vi "about.vi"() -> ()   [LabVIEW 2014]
panel:
  out "专利信息":string
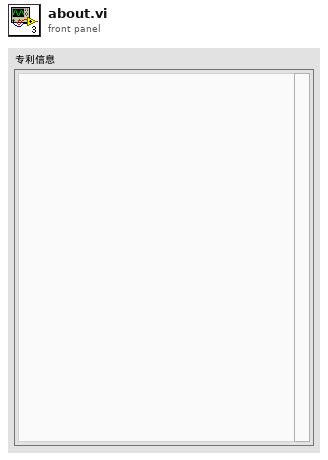
[diagram p1: front panel]
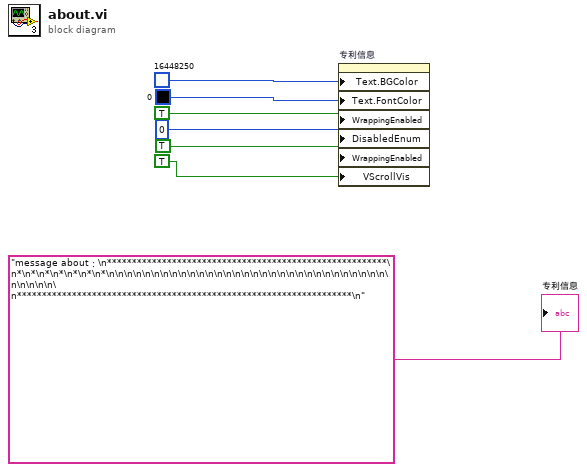
[diagram p0: block diagram]
diagram:
  n1 = property on="专利信息" class="Str"("Text.BGColor"=u32 16448250, "Text.FontColor"=u32 0, "WrappingEnabled"=TRUE, "DisabledEnum"=0, "WrappingEnabled"=TRUE, "VScrollVis"=TRUE) -> ()  [unwired: 2 in, 2 out]
  "专利信息" <- "message about：\n********************************************************\n*\n*\n*\n*\n*\n*\n*\n\n\n\n\n\n\n\n\n\n\n\n\n\n\n\n\n\n\n\n\n\n\n\n\n\n\n\n\n\n\n\n\n\n\n\n\n*******************************************************************\n"
